vi "Get Column Path.vi"(8 "error in (no error)":errorcluster, 9 "Column":string, 10 "Table path":string, 11 "Data.PG in":refnum<class "Data.PGSQL.lvclass">) -> (0 "error out":errorcluster, 1 "Column Unit":string, 2 "Column Path":string, 3 "Data.PG out":refnum<class "Data.PGSQL.lvclass">)   [LabVIEW 2013, in "Data.PGSQL.lvclass"]
uses:
  Data.PGSQL.lvclass
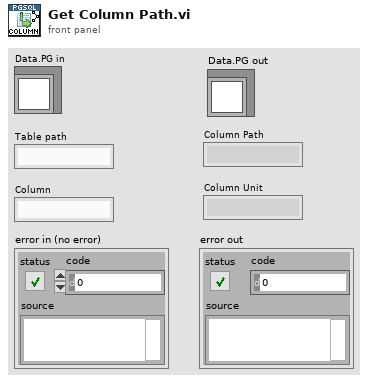
[diagram p1: front panel]
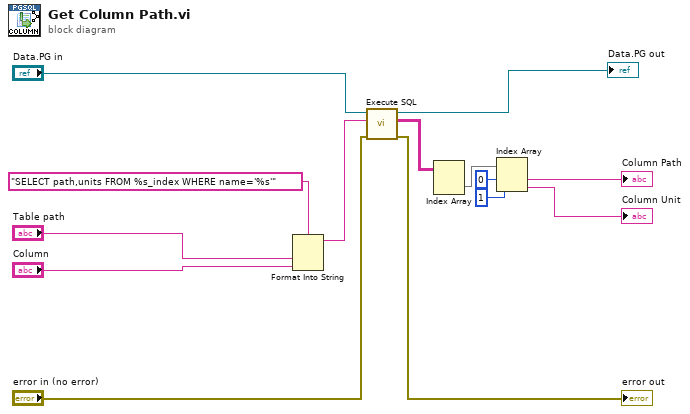
[diagram p0: block diagram]
diagram:
  n1 = Format Into String(format string="SELECT path,units FROM %s_index WHERE name='%s'", "Table path", "Column") -> (resulting string=w4:string)  [unwired: 2 in, 1 out]
  n2 = call "Execute SQL.vi"("error in"="error in (no error)", "SQL"=w4, "Data.PG"="Data.PG in") -> ("error out"=→"error out":errorcluster, "Result"=w5:string[][], "Data.PG out"=→"Data.PG out":refnum<class "Data.PGSQL.lvclass">)  [unwired: 6 in]
  n3 = Index Array(array=w5) -> (element=w6:string[])  [unwired: 2 in]
  n4 = Index Array(array=w6, index #1=0 ("index"), index #2=1 ("index")) -> (element #1=→"Column Path":string, element #2=→"Column Unit":string)
